vi "index.vi"() -> ()   [LabVIEW 2025]
uses:
  <vilib>/Analysis/3filter.llb/Filter Passband Type.ctl
  <vilib>/measure/maspectr.llb/FFT Spectrum (Mag-Phase) for 1 Chan.vi
  <vilib>/measure/NI_MAPro.lvlib
  <vilib>/Analysis/NI_AALBase.lvlib
panel:
  out "iterace":dbl
  in  "Stop":bool
  in  "Tab Control":T1(tab)
  out "Waveform Graph 2":cluster{"f0":dbl, "df":dbl, "magnitude":dbl[]}(graph)
  out "Počet BPM":dbl
  in  "hint":bool
  in  "loadSignal":bool
  out "Waveform Graph":waveform(dbl)(graph)
  out "graf EMG":waveform(dbl)(graph)
  in  "load EMG":bool
  out "Spektrum EMG":cluster{"f0":dbl, "df":dbl, "magnitude":dbl[]}(graph)
  in  "load EEG":bool
  out "EEG graf":waveform(dbl)(graph)
  out "Waveform Graph 4":cluster{"f0":dbl, "df":dbl, "magnitude":dbl[]}(graph)
  # "Aplikace pro laboratorní měření biosignálů"
  # "Úloha č. 1: Měření a analýza EKG signálu"
  # "Úloha č. 2: Měření a analýza EMG signálu"
  # "Úloha č. 3: Měření a analýza EEG signálu"
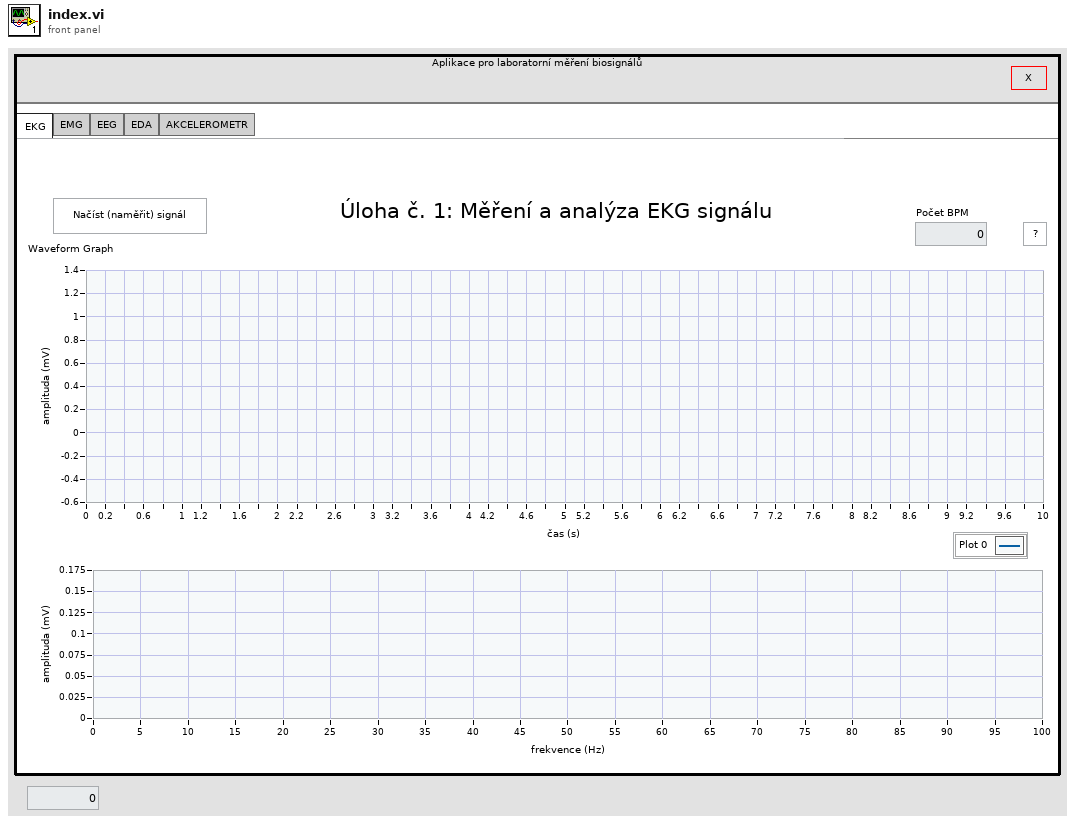
[diagram p1: front panel]
types:
  T1 = enum32{" EKG", "EMG", "EEG", "EDA", "AKCELEROMETR"}
  T2 = typedef "NI_AALBase.lvlib/Filter Passband Type.ctl" = enum32{"Lowpass", "Highpass", "Bandpass", "Bandstop"}
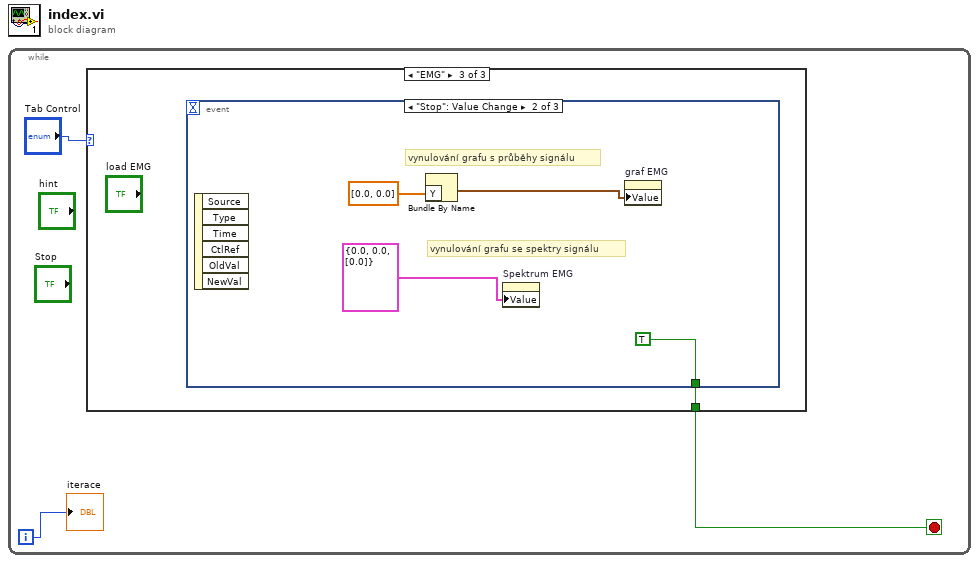
[diagram p0: block diagram]
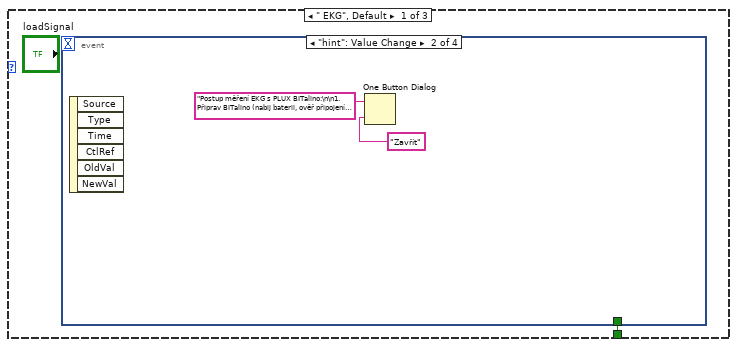
[diagram p2: hidden frame]
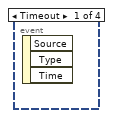
[diagram p3: hidden frame]
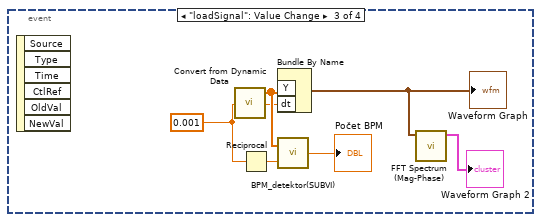
[diagram p4: hidden frame]
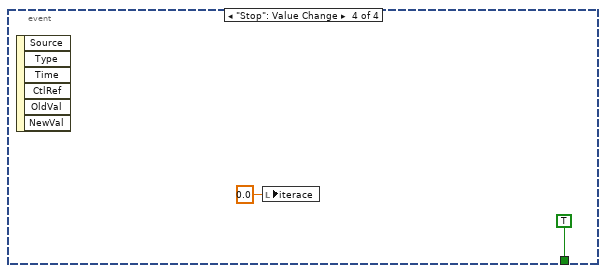
[diagram p5: hidden frame]
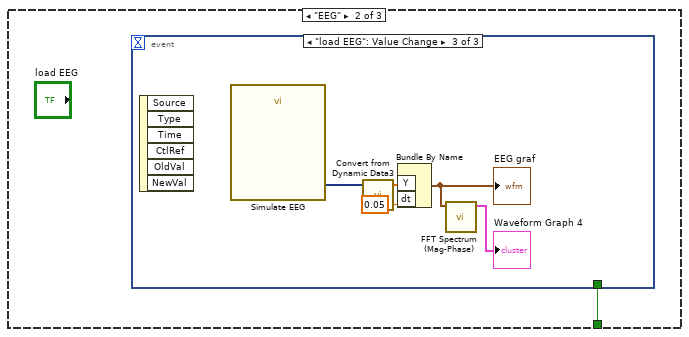
[diagram p6: hidden frame]
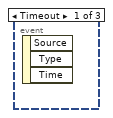
[diagram p7: hidden frame]
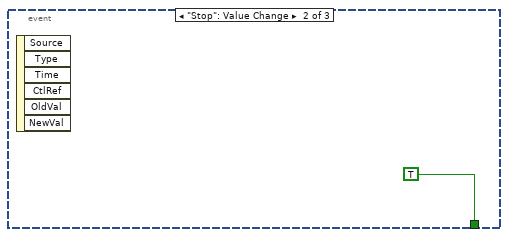
[diagram p8: hidden frame]
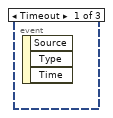
[diagram p9: hidden frame]
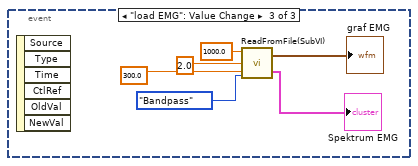
[diagram p10: hidden frame]
diagram:
  n1 = while {
    i -> [w1]
    stop <- w2 stop-if-true
    n2 = case shown="\"EMG\"" "Tab Control" {
      tunnel: [w4 w15 w22] -> w2
      frame " EKG", Default {
        n3 = event shown="[1] \"hint\": Value Change" {
          selector: _ -> [_ _ _ _]
          dyn-events: _ -> [_ _ _ _]
          timeout: _ -> [_ _ _ _]
          tunnel: [_ _ _ TRUE] -> w4
          event Timeout {
            n4 = event-data() -> ()  [unwired: 1 in, 3 out]
          }
          event "hint": Value Change {
            n5 = event-data() -> ()  [unwired: 1 in, 6 out]
            n6 = One Button Dialog(message="Postup měření EKG s PLUX BITalino:\n\n1. Připrav BITalino (nabij baterii, ověř připojení).\n2. Očisti kůži v místě nalepení elektrod alkoholem.\n3. Přilep první elektrodu pod pravou klíční kost.\n4. Přilep druhou elektrodu na levý bok hrudníku, pod srdcem.\n5. Přilep třetí referenční elektrodu na pravý dolní hrudník nebo bok.\n6. Propoj elektrody s EKG vstupem BITalino.\n7. Zkontroluj kvalitu signálu a případně uprav elektrody.\n", button name ("OK")="Zavřít") -> ()  [unwired: 1 out]
          }
          event "loadSignal": Value Change {
            w10 = 0.001 ("dt")
            n7 = event-data() -> ()  [unwired: 1 in, 6 out]
            n8 = call "Convert from Dynamic Data"() -> ("Array"=w12:dbl[])  [unwired: 4 in]
            n9 = Reciprocal(x=w10) -> (1/x=w11:dbl)
            n10 = Bundle By Name("Y"=w12, "dt"=w10) -> (w8:waveform(dbl))  [unwired: 1 in]
            "Waveform Graph" <- w8
            n11 = call "BPM_detektor(SUBVI).vi"("Vzorkovacka"=w11, "Vstupní signál"=w12) -> ("Hodnota BPM"=→"Počet BPM":dbl)
            n12 = call-poly <vilib>:"FFT Spectrum (Mag-Phase).vi"("time signal"=w8) -> ("magnitude"=→"Waveform Graph 2":cluster{"f0":dbl, "df":dbl, "magnitude":dbl[]})  [unwired: 6 in, 4 out]
          }
          event "Stop": Value Change {
            n13 = event-data() -> ()  [unwired: 1 in, 6 out]
            n14 = local write "iterace"(0.0 ("iterace")) -> ()
          }
        }
      }
      frame "EEG" {
        n15 = event shown="[2] \"load EEG\": Value Change" {
          selector: _ -> [_ _ _]
          dyn-events: _ -> [_ _ _]
          timeout: _ -> [_ _ _]
          tunnel: [_ TRUE _] -> w15
          event Timeout {
            n16 = event-data() -> ()  [unwired: 1 in, 3 out]
          }
          event "Stop": Value Change {
            n17 = event-data() -> ()  [unwired: 1 in, 6 out]
          }
          event "load EEG": Value Change {
            n18 = event-data() -> ()  [unwired: 1 in, 6 out]
            n19 = call "Simulate EEG"() -> ("EEG"=w21:dynamicdata)  [unwired: 10 in, 1 out]
            n20 = call "Convert from Dynamic Data3"("Dynamic Data Type"=w21) -> ("Array"=w20:dbl[])  [unwired: 3 in]
            n21 = Bundle By Name("Y"=w20, "dt"=0.05) -> (w18:waveform(dbl))  [unwired: 1 in]
            "EEG graf" <- w18
            n22 = call-poly <vilib>:"FFT Spectrum (Mag-Phase).vi"("time signal"=w18) -> ("magnitude"=→"Waveform Graph 4":cluster{"f0":dbl, "df":dbl, "magnitude":dbl[]})  [unwired: 6 in, 4 out]
          }
        }
      }
      frame "EMG" {
        n23 = event shown="[1] \"Stop\": Value Change" {
          selector: _ -> [_ _ _]
          dyn-events: _ -> [_ _ _]
          timeout: _ -> [_ _ _]
          tunnel: [_ TRUE _] -> w22
          event Timeout {
            n24 = event-data() -> ()  [unwired: 1 in, 3 out]
          }
          event "Stop": Value Change {
            # "vynulování grafu se spektry signálu"
            # "vynulování grafu s průběhy signálu"
            n25 = event-data() -> ()  [unwired: 1 in, 6 out]
            n26 = Bundle By Name("Y"=dbl[] [0.0, 0.0]) -> (w23:waveform(dbl))  [unwired: 1 in]
            n27 = property on="Spektrum EMG" class="WFGraph (strict)"("Value"=cluster{"f0":dbl, "df":dbl, "magnitude":dbl[]} {"f0"=0.0, "df"=0.0, "magnitude"=[0.0]} ("Spektrum")) -> ()  [unwired: 2 in, 2 out]
            n28 = property on="graf EMG" class="WFGraph (strict)"("Value"=w23) -> ()  [unwired: 2 in, 2 out]
          }
          event "load EMG": Value Change {
            n29 = event-data() -> ()  [unwired: 1 in, 6 out]
            n30 = call "ReadFromFile(SubVI).vi"("filter type"=Filter_Passband_Type."Bandpass", "Horni Mezni Frekvence (Hz)"=300.0, "Dolni Mezni Frekvence (Hz)"=2.0, "Sampling Freq"=1000.0) -> ("Amplitudove Spektrum"=→"Spektrum EMG":cluster{"f0":dbl, "df":dbl, "magnitude":dbl[]}, "Waveform Graf"=→"graf EMG":waveform(dbl))
          }
        }
      }
    }
    "iterace" <- w1
  }
